vi "Find_Place_of_Missed_Point-1.vi"(4 "[IN] Index of problem\ndisplacement inside track":i32, 5 "[IN] Time Point of Mi\nssed Problem Dot":i32, 6 "error IN":errorcluster, 7 "[IN] Dot Status":i16, 8 "[IN] Missed track":dbl[](array[numeric]), 9 "[IN] Track group":T1) -> (0 "error OUT":errorcluster, 2 "[OUT] Index of \nconnected dots\ninside the track":i32[](array[numeric]), 3 "[OUT] Index of connected\ntracks with problem dot":i32[](array[numeric]))   [LabVIEW 2013]
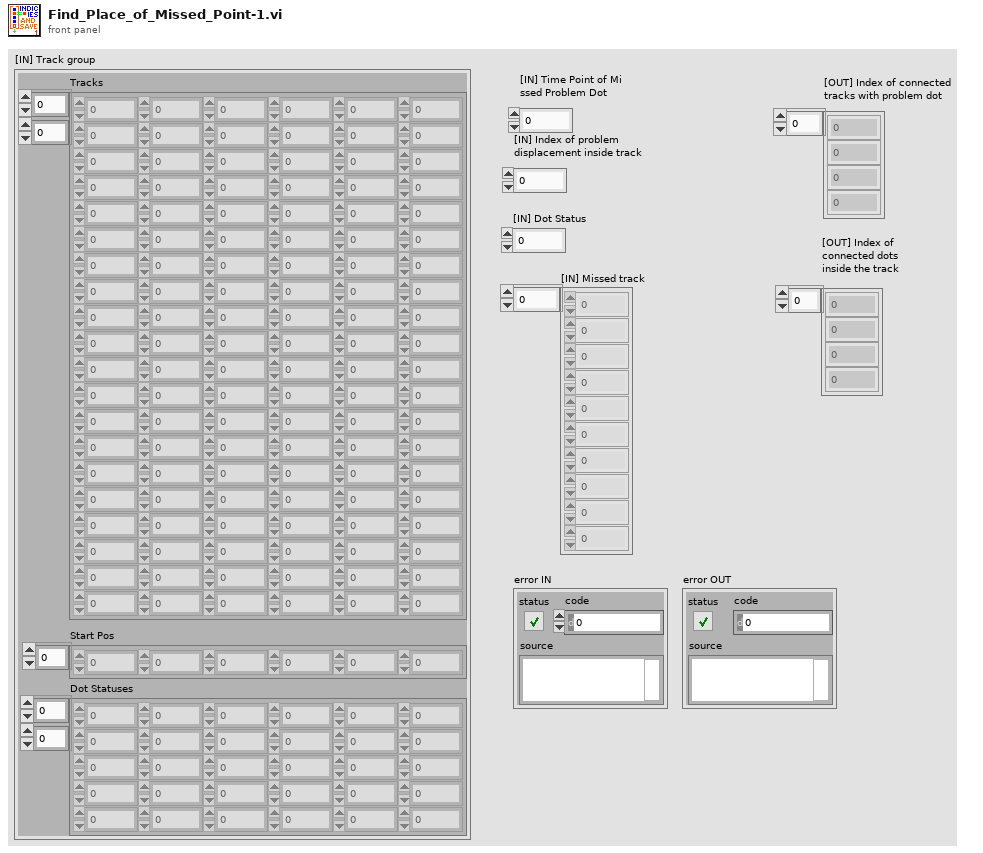
[diagram p1: front panel]
types:
  T1 = cluster{"Tracks":dbl[][], "Start Pos":i32[], "Dot Statuses":i16[][]}
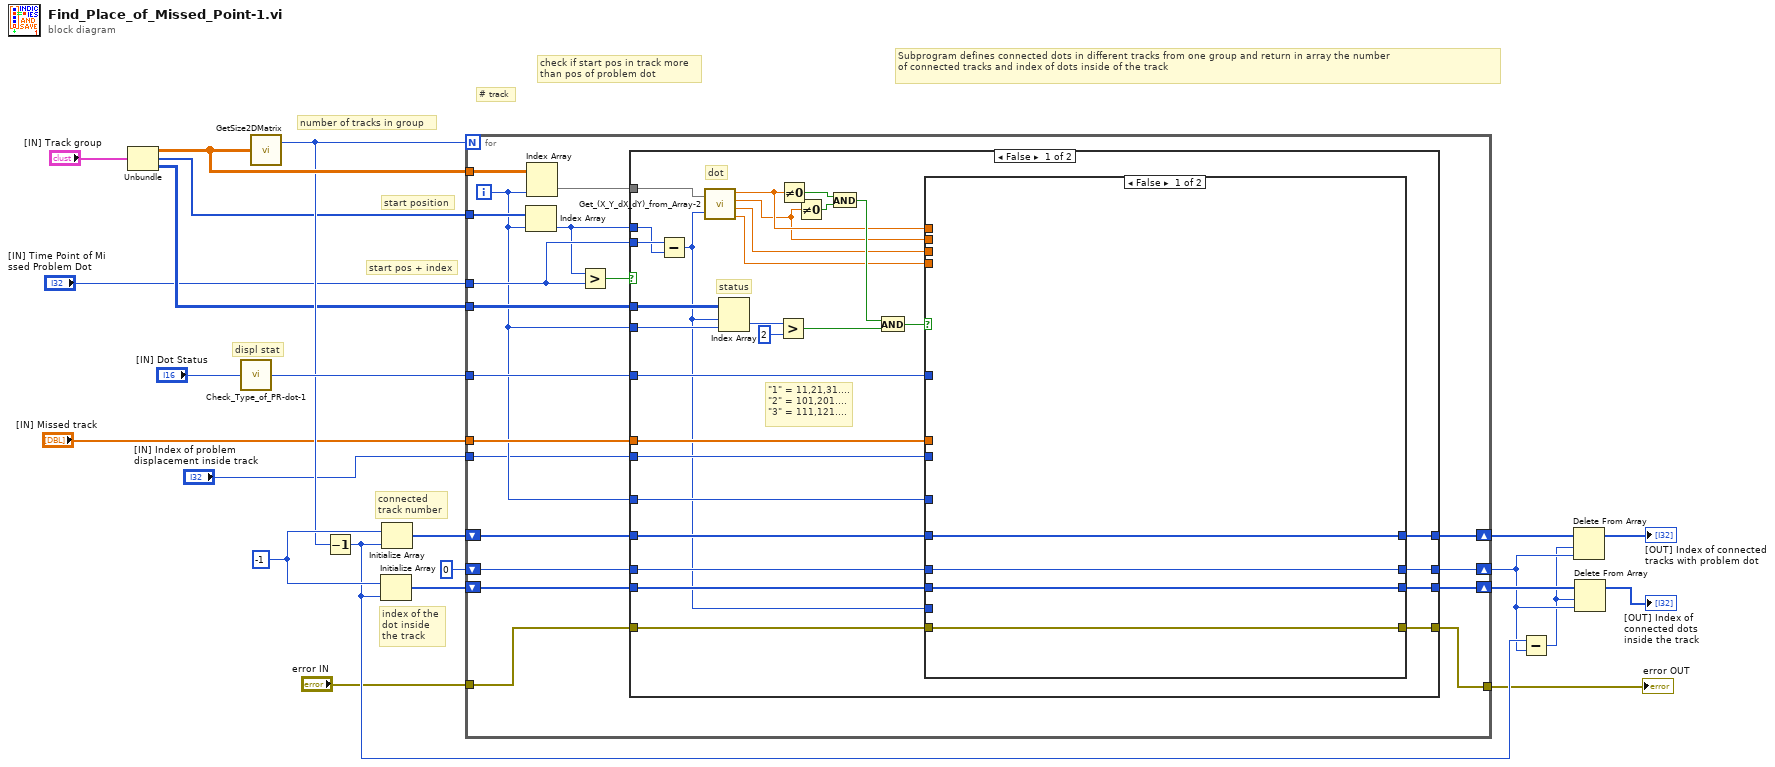
[diagram p0: block diagram]
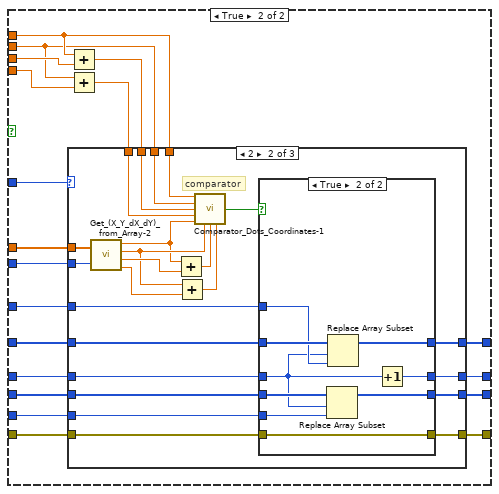
[diagram p2: hidden frame]
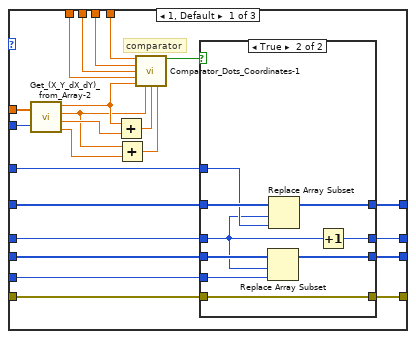
[diagram p3: hidden frame]
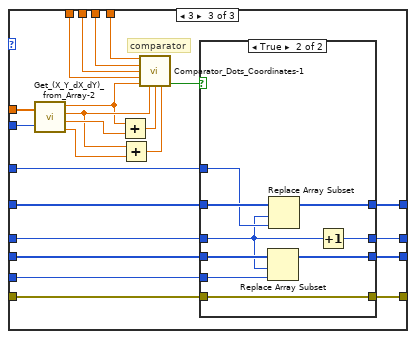
[diagram p6: hidden frame]
diagram:
  w20 = -1 ("disabled index (row)")
  # "start pos + index"
  # "Subprogram defines connected dots in different tracks from one group and return in array the number\nof connected tracks and index of dots inside of the track"
  # "# track"
  # "start position"
  # "number of tracks in group"
  # "check if start pos in track more \nthan pos of problem dot"
  # "index of the dot inside \nthe track"
  # "connected\ntrack number"
  # "displ stat"
  n1 = Unbundle("[IN] Track group") -> ("Tracks"=w22:dbl[][], "Start Pos"=w15:i32[], "Dot Statuses"=w14:i16[][])
  n2 = call "Check_Type_of_PR-dot-1.vi"("[IN] dot status"="[IN] Dot Status") -> ("[OUT] Type of\nproblem dot"=w21:i32)
  n3 = call "GetSize2DMatrix.vi"("Array IN (2D)"=w22) -> ("# Cols"=w19:i32)  [unwired: 1 out]
  n4 = Decrement(x=w19) -> (x-1=w12:i32)
  n5 = Initialize Array(w20, w12) -> (w17:i32[])
  n6 = Initialize Array(w20, w12) -> (w18:i32[])
  n7 = for {
    N: w19 -> [_]
    tunnel: w22 -> [w42]
    tunnel: w21 -> [w38]
    tunnel: "[IN] Time Point of Mi\nssed Problem Dot" -> [w39]
    shift-right: [w32] -> w13
    shift-left: w18 -> [w41]
    shift-right: [w30] -> w11
    shift-left: w17 -> [w40]
    shift-right: [w31] -> w10
    shift-left: 0 -> [w37]
    tunnel: w15 -> [w36]
    tunnel: w14 -> [w35]
    tunnel: "[IN] Missed track" -> [w34]
    tunnel: "error IN" -> [w29]
    tunnel: [w28] -> w5
    tunnel: "[IN] Index of problem\ndisplacement inside track" -> [w24]
    i -> [w33]
    n8 = Index Array(array=w36, index=w33) -> (element=w25:i32)
    n9 = Index Array(array=w42, index (col)=w33) -> (element=w26:dbl[])  [unwired: 1 in]
    n10 = Greater?(x=w25, y=w39) -> (0:w27:bool)
    n11 = case shown="False" w27 {
      tunnel: w26 -> [w53 _]
      tunnel: w25 -> [w49 _]
      tunnel: w39 -> [w50 _]
      tunnel: w35 -> [w69 _]
      tunnel: w33 -> [w68 _]
      tunnel: w38 -> [w64 _]
      tunnel: w34 -> [w63 _]
      tunnel: w41 -> [w62 w206]
      tunnel: w37 -> [w61 w205]
      tunnel: w40 -> [w60 w204]
      tunnel: w33 -> [w59 _]
      tunnel: [w58 w206] -> w32
      tunnel: [w57 w205] -> w31
      tunnel: [w56 w204] -> w30
      tunnel: w29 -> [w55 w203]
      tunnel: [w54 w203] -> w28
      tunnel: w24 -> [w48 _]
      frame False {
        # "\"1\" = 11,21,31....\n\"2\" = 101,201....\n\"3\" = 111,121...."
        # "status"
        # "dot"
        n12 = Subtract(x=w50, y=w49) -> (x-y=w45:i32)
        n13 = call "Get_(X_Y_dX_dY)_from_Array-2.vi"("(X,Y,dX,dY)"=w53, "Index of Displacement"=w45) -> ("X"=w52:dbl, "Y"=w51:dbl, "dX"=w47:dbl, "dY"=w46:dbl)
        n14 = Index Array(array=w69, index (row)=w45, index (col)=w68) -> (element=w67:i16)
        n15 = Greater?(x=w67, y=i16 2) -> (0:w44:bool)
        n16 = Not Equal To 0?(x=w52) -> (x != 0?=w70:bool)
        n17 = Not Equal To 0?(x=w51) -> (x != 0?=w71:bool)
        n18 = And(x=w70, y=w71) -> (x .and. y?=w65:bool)
        n19 = And(x=w65, y=w44) -> (x .and. y?=w43:bool)
        n20 = case shown="False" w43 {
          tunnel: w64 -> [_ w94]
          tunnel: w52 -> [_ w90]
          tunnel: w51 -> [_ w89]
          tunnel: w47 -> [_ w92]
          tunnel: w46 -> [_ w91]
          tunnel: w63 -> [_ w93]
          tunnel: w62 -> [w75 w86]
          tunnel: w61 -> [w74 w85]
          tunnel: w60 -> [w73 w84]
          tunnel: w59 -> [_ w83]
          tunnel: w45 -> [_ w82]
          tunnel: [w75 w81] -> w58
          tunnel: [w74 w80] -> w57
          tunnel: [w73 w79] -> w56
          tunnel: w55 -> [w72 w78]
          tunnel: [w72 w77] -> w54
          tunnel: w48 -> [_ w76]
          frame False {
          }
          frame True {
            n21 = Add(x=w90, y=w92) -> (x+y=w88:dbl)
            n22 = Add(x=w89, y=w91) -> (x+y=w87:dbl)
            n23 = case shown="2" w94 {
              tunnel: w93 -> [w102 w136 w172]
              tunnel: w90 -> [w117 w150 w186]
              tunnel: w89 -> [w116 w151 w187]
              tunnel: w88 -> [w115 w152 w188]
              tunnel: w87 -> [w114 w153 w189]
              tunnel: w86 -> [w112 w147 w184]
              tunnel: w85 -> [w111 w146 w183]
              tunnel: w84 -> [w110 w145 w182]
              tunnel: w83 -> [w109 w148 w185]
              tunnel: w82 -> [w108 w144 w181]
              tunnel: [w107 w143 w180] -> w81
              tunnel: [w106 w142 w179] -> w80
              tunnel: [w105 w141 w178] -> w79
              tunnel: w78 -> [w104 w140 w176]
              tunnel: [w103 w139 w175] -> w77
              tunnel: w76 -> [w101 w135 w171]
              frame 1, Default {
                # "comparator"
                n24 = call "Get_(X_Y_dX_dY)_from_Array-2.vi"("(X,Y,dX,dY)"=w102, "Index of Displacement"=w101) -> ("X"=w100:dbl, "Y"=w97:dbl, "dX"=w99:dbl, "dY"=w96:dbl)
                n25 = Add(x=w100, y=w99) -> (x+y=w98:dbl)
                n26 = Add(x=w97, y=w96) -> (x+y=w95:dbl)
                n27 = call "Comparator_Dots_Coordinates-1.vi"("X1"=w117, "Y1"=w116, "(X+dX)1"=w115, "(Y+dY)1"=w114, "X2"=w100, "Y2"=w97, "(X+dX)2"=w98, "(Y+dY)2"=w95) -> ("X1=X2,Y1=Y2 (1)"=w113:bool)  [unwired: 5 in, 2 out]
                n28 = case shown="True" w113 {
                  tunnel: w112 -> [w121 w130]
                  tunnel: w111 -> [w120 w126]
                  tunnel: w110 -> [w119 w128]
                  tunnel: w109 -> [_ w129]
                  tunnel: w108 -> [_ w127]
                  tunnel: [w121 w125] -> w107
                  tunnel: [w120 w124] -> w106
                  tunnel: [w119 w123] -> w105
                  tunnel: [w118 w122] -> w103
                  tunnel: w104 -> [w118 w122]
                  frame False {
                  }
                  frame True {
                    n29 = Replace Array Subset(array=w128, new element=w127, index=w126) -> (w123:i32[])
                    n30 = Replace Array Subset(array=w130, new element=w129, index=w126) -> (w125:i32[])
                    n31 = Increment(x=w126) -> (x+1=w124:i32)
                  }
                }
              }
              frame 2 {
                # "comparator"
                n32 = call "Get_(X_Y_dX_dY)_from_Array-2.vi"("(X,Y,dX,dY)"=w136, "Index of Displacement"=w135) -> ("X"=w131:dbl, "Y"=w134:dbl, "dX"=w138:dbl, "dY"=w137:dbl)
                n33 = Add(x=w131, y=w138) -> (x+y=w133:dbl)
                n34 = Add(x=w134, y=w137) -> (x+y=w132:dbl)
                n35 = call "Comparator_Dots_Coordinates-1.vi"("X1"=w150, "Y1"=w151, "(X+dX)1"=w152, "(Y+dY)1"=w153, "X2"=w131, "Y2"=w134, "(X+dX)2"=w133, "(Y+dY)2"=w132) -> ("X1(2)=X2(2),Y1(2)=Y2(2) (2)"=w149:bool)  [unwired: 5 in, 2 out]
                n36 = case shown="True" w149 {
                  tunnel: w147 -> [w157 w166]
                  tunnel: w146 -> [w156 w162]
                  tunnel: w145 -> [w155 w164]
                  tunnel: w148 -> [_ w165]
                  tunnel: w144 -> [_ w163]
                  tunnel: [w157 w161] -> w143
                  tunnel: [w156 w160] -> w142
                  tunnel: [w155 w159] -> w141
                  tunnel: w140 -> [w154 w158]
                  tunnel: [w154 w158] -> w139
                  frame False {
                  }
                  frame True {
                    n37 = Replace Array Subset(array=w164, new element=w163, index=w162) -> (w159:i32[])
                    n38 = Replace Array Subset(array=w166, new element=w165, index=w162) -> (w161:i32[])
                    n39 = Increment(x=w162) -> (x+1=w160:i32)
                  }
                }
              }
              frame 3 {
                # "comparator"
                n40 = call "Get_(X_Y_dX_dY)_from_Array-2.vi"("(X,Y,dX,dY)"=w172, "Index of Displacement"=w171) -> ("X"=w167:dbl, "Y"=w170:dbl, "dX"=w174:dbl, "dY"=w173:dbl)
                n41 = Add(x=w167, y=w174) -> (x+y=w168:dbl)
                n42 = Add(x=w170, y=w173) -> (x+y=w169:dbl)
                n43 = call "Comparator_Dots_Coordinates-1.vi"("X1"=w186, "Y1"=w187, "(X+dX)1"=w188, "(Y+dY)1"=w189, "X2"=w167, "Y2"=w170, "(X+dX)2"=w168, "(Y+dY)2"=w169) -> ("(1) OR (2) = (3)"=w177:bool)  [unwired: 5 in, 2 out]
                n44 = case shown="True" w177 {
                  tunnel: w184 -> [w193 w202]
                  tunnel: w183 -> [w192 w198]
                  tunnel: w182 -> [w191 w200]
                  tunnel: w185 -> [_ w201]
                  tunnel: w181 -> [_ w199]
                  tunnel: [w193 w197] -> w180
                  tunnel: [w192 w196] -> w179
                  tunnel: [w191 w195] -> w178
                  tunnel: w176 -> [w190 w194]
                  tunnel: [w190 w194] -> w175
                  frame False {
                  }
                  frame True {
                    n45 = Replace Array Subset(array=w200, new element=w199, index=w198) -> (w195:i32[])
                    n46 = Replace Array Subset(array=w202, new element=w201, index=w198) -> (w197:i32[])
                    n47 = Increment(x=w198) -> (x+1=w196:i32)
                  }
                }
              }
            }
          }
        }
      }
      frame True {
      }
    }
  }
  "error OUT" <- w5
  n48 = Subtract(x=w12, y=w10) -> (x-y=w9:i32)
  n49 = Delete From Array(array=w13, length=w9, index=w10) -> (array with subset deleted=→"[OUT] Index of connected\ntracks with problem dot":i32[])  [unwired: 1 out]
  n50 = Delete From Array(array=w11, length=w9, index=w10) -> (array with subset deleted=→"[OUT] Index of \nconnected dots\ninside the track":i32[])  [unwired: 1 out]
